vi "MCP23S17 SYS Port A Set.vi"(8 "error in (no error)":errorcluster, 9 "Channels":u16 max=1023, 10 "Addr":T1 items=["Addr-0"=0, "Addr-1"=4, "Addr-2"=2, "Addr-3"=6, "Addr-4"=1, "Addr-5"=5, "Addr-6"=3, "Addr-7"=7], 11 "handle":u32 format="%08x") -> (0 "error out":errorcluster, 3 "handle out":u32)   [LabVIEW 2018]
uses:
  PROJEKT/NIKO/Labview/Niko V4/FTDI SPI/Ctl/Sub Addr.ctl
  PROJEKT/NIKO/Labview/Niko V5/FTDI SPI/libMPSSE-SPI.lvlib
panel:
  out "string 4":string
  out "string 3":string
  out "string 2":string
  out "string":string
  in  "Array U8":u8[](array[numeric])=[64, 18, 0, 128, 0, 0, 0, 0, 0, 0] format="%x"
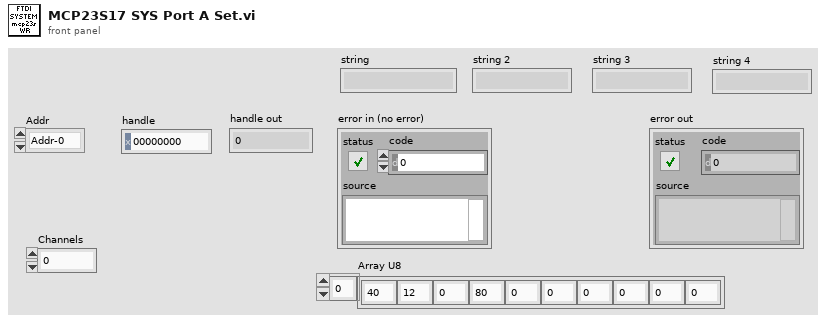
[diagram p1: front panel]
types:
  T1 = typedef "Sub Addr.ctl" = u16
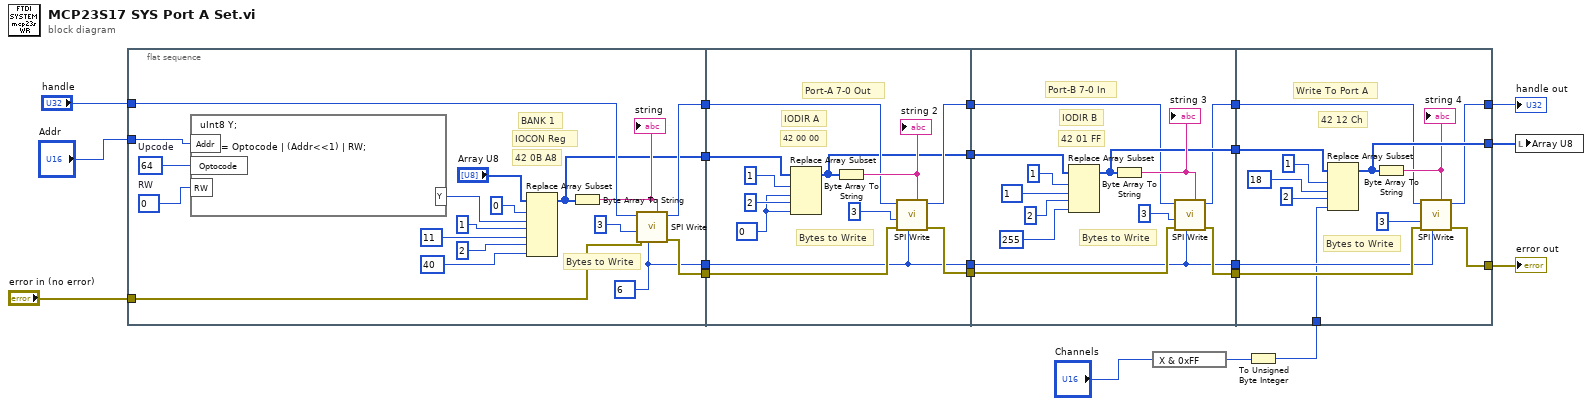
[diagram p0: block diagram]
diagram:
  n1 = flat-sequence {
    tunnel: "Addr" -> [w38]
    tunnel: "handle" -> [w32]
    tunnel: [w30] -> w21
    tunnel: [w29] -> w20
    tunnel: [w28] -> w19
    tunnel: [w27] -> w18
    tunnel: "error in (no error)" -> [w26]
    tunnel: w21 -> [w50]
    tunnel: w20 -> [w44]
    tunnel: w19 -> [w48]
    tunnel: w18 -> [w41]
    tunnel: [w49] -> w17
    tunnel: [w43] -> w16
    tunnel: [w42] -> w15
    tunnel: [w41] -> w14
    tunnel: w17 -> [w59]
    tunnel: w16 -> [w57]
    tunnel: w15 -> [w61]
    tunnel: w14 -> [w53]
    tunnel: [w58] -> w13
    tunnel: [w56] -> w12
    tunnel: [w60] -> w11
    tunnel: [w53] -> w4
    tunnel: [w74] -> w6
    tunnel: [w76] -> w8
    tunnel: [w71] -> w7
    tunnel: w13 -> [w72]
    tunnel: w12 -> [w77]
    tunnel: w11 -> [w75]
    tunnel: w10 -> [w65]
    tunnel: w4 -> [w66]
    frame #0 {
      w22 = u8 64  # Upcode
      w23 = u8 0  # RW
      w27 = u8 6
      # "BANK 1"
      # "IOCON Reg"
      # "Bytes to Write"
      # "42 0B A8"
      n2 = formula code="uInt8 Y;\n      \n    Y = Optocode | (Addr<<1) | RW;"("Addr"=w38, "Optocode"=w22, "RW"=w23) -> ("Y"=w37:u8)
      n3 = Replace Array Subset(array="Array U8", new element #1=w37, index #1=0 ("index"), new element #2=u8 11, index #2=u8 1 ("new element/subarray"), new element #3=u8 40, index #3=2 ("index")) -> (w28:u8[])
      n4 = Byte Array To String(unsigned byte array=w28) -> (string=w31:string)
      "string" <- w31
      n5 = call "SPI Write.vi"("buffer"=w31, "options"=w27, "error in (no error)"=w26, "Bytes To Send"=u32 3, "handle"=w32) -> ("error out"=w29:errorcluster, "handle out"=w30:u32)  [unwired: 4 in, 1 out]
    }
    frame #1 {
      w45 = u8 0
      # "IODIR A"
      # "Port-A 7-0 Out"
      # "Bytes to Write"
      # "42 00 00"
      n6 = Replace Array Subset(array=w48, new element #1=w45, index #1=1 ("index"), new element #2=w45, index #2=2 ("index")) -> (w42:u8[])
      n7 = Byte Array To String(unsigned byte array=w42) -> (string=w51:string)
      "string 2" <- w51
      n8 = call "SPI Write.vi"("buffer"=w51, "options"=w41, "error in (no error)"=w44, "Bytes To Send"=u32 3, "handle"=w50) -> ("error out"=w43:errorcluster, "handle out"=w49:u32)  [unwired: 4 in, 1 out]
    }
    frame #2 {
      # "IODIR B"
      # "Port-B 7-0 In"
      # "Bytes to Write"
      # "42 01 FF"
      n9 = Replace Array Subset(array=w61, new element #1=u8 1, index #1=1 ("index"), new element #2=u8 255, index #2=2 ("index")) -> (w60:u8[])
      n10 = Byte Array To String(unsigned byte array=w60) -> (string=w62:string)
      "string 3" <- w62
      n11 = call "SPI Write.vi"("buffer"=w62, "options"=w53, "error in (no error)"=w57, "Bytes To Send"=u32 3, "handle"=w59) -> ("error out"=w56:errorcluster, "handle out"=w58:u32)  [unwired: 4 in, 1 out]
    }
    frame #3 {
      # "Write To Port A"
      # "Bytes to Write"
      # "42 12 Ch"
      n12 = Replace Array Subset(array=w75, new element #1=u8 18, index #1=1 ("index"), new element #2=w65, index #2=2 ("index")) -> (w74:u8[])
      n13 = Byte Array To String(unsigned byte array=w74) -> (string=w73:string)
      "string 4" <- w73
      n14 = call "SPI Write.vi"("buffer"=w73, "options"=w66, "error in (no error)"=w77, "Bytes To Send"=u32 3, "handle"=w72) -> ("error out"=w76:errorcluster, "handle out"=w71:u32)  [unwired: 4 in, 1 out]
    }
  }
  n15 = expression code="X & 0xFF"("Channels") -> (w2:u16)
  n16 = To Unsigned Byte Integer(number=w2) -> (unsigned 8bit integer=w10:u8)
  n17 = local write "Array U8"(w6) -> ()
  "error out" <- w8
  "handle out" <- w7
